vi "Player Info.vi"(11 "Voyager in":refnum<class "Voyager.lvclass">) -> (0 "Defeat Speech":string, 1 "Victory Speech":string, 2 "Name":string, 3 "Voyager out":refnum<class "Voyager.lvclass">)   [LabVIEW 2015, in "Voyager.lvclass"]
uses:
  Voyager.lvclass
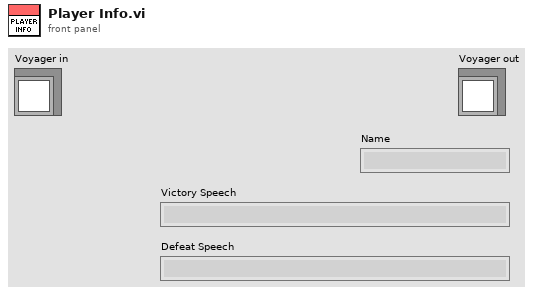
[diagram p1: front panel]
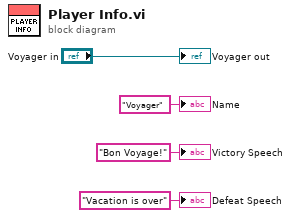
[diagram p0: block diagram]
diagram:
  "Voyager out" <- "Voyager in"
  "Name" <- "Voyager" ("Name")
  "Victory Speech" <- "Bon Voyage!" ("Victory Speech")
  "Defeat Speech" <- "Vacation is over" ("Defeat Speech")
